vi "Send user input.vi"(7 "Milk intensity":dbl, 8 "error in":errorcluster, 9 "Coffe intensity":dbl, 10 "Choose Coffee":string(combo)) -> (0 "error out":errorcluster)   [LabVIEW 2024, in "Coffee Prefers.lvlib"]
doc: "Send selections to other models\n_____\nCreated using DQMH Event Scripter 7.0.1.1316."
uses:
  Coffee Prefers.lvlib
  Send user input Argument--cluster.ctl
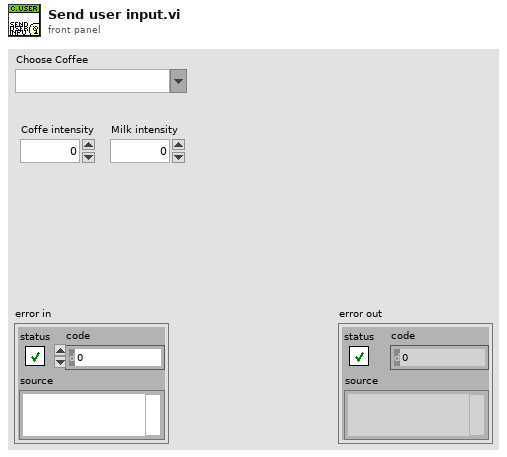
[diagram p1: front panel]
types:
  T1 = typedef "Coffee Prefers.lvlib/Send user input Argument--cluster.ctl" = cluster{"Coffe intensity":dbl, "Milk intensity":dbl, "Choose Coffe":string}
  T2 = typedef "Coffee Prefers.lvlib/Broadcast Events--cluster.ctl" = cluster{"Module Did Init":refnum<user-event>, "Status Updated":refnum<user-event>, "Error Reported":refnum<user-event>, "Module Did Stop":refnum<user-event>, "Update Module Execution Status":refnum<user-event>, "Send user input":refnum<user-event>}
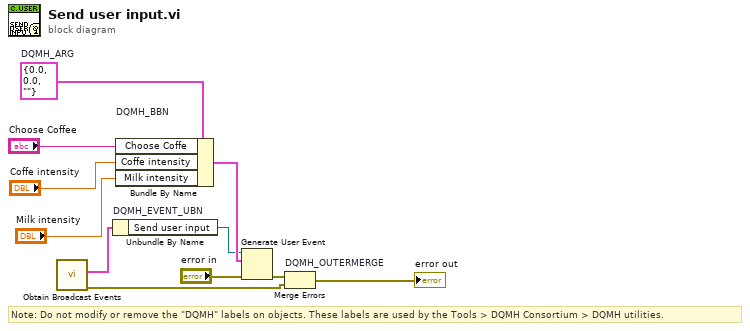
[diagram p0: block diagram]
diagram:
  w6 = T1 {"Coffe intensity"=0.0, "Milk intensity"=0.0, "Choose Coffe"=""}  # DQMH_ARG
  # "Note: Do not modify or remove the \"DQMH\" labels on objects. These labels are used by the Tools > DQMH Consortium > DQMH utilities."
  n1 = call "Obtain Broadcast Events.vi"() -> ("error out"=w2:errorcluster, "Coffee Prefers Broadcast Events"=w1:T2)  [unwired: 10 in]
  n2 = Unbundle By Name "DQMH_EVENT_UBN"(w1) -> ("Send user input"=w8:refnum<user-event>)
  n3 = Bundle By Name "DQMH_BBN"(cluster=w6, "Choose Coffe"="Choose Coffee", "Coffe intensity"="Coffe intensity", "Milk intensity"="Milk intensity") -> (w9:T1)
  n4 = Generate User Event(user event=w8, event data cluster=w9, error in="error in") -> (error out=w7:errorcluster)  [unwired: 1 in, 1 out]
  n5 = Merge Errors "DQMH_OUTERMERGE"(w7, w2) -> (→"error out":errorcluster)
